vi "Find_Serial_Port.vi"(8 "error in":errorcluster) -> (0 "error out":errorcluster, 3 "Array":string[](array[string]))   [LabVIEW 2011]
doc: "This VI finds the VISA Resource Names of all COM ports on the host machine. It first finds the VISA Resource Names of all serial ports and then filters through these to find which of those are COM ports."
panel:
  out "Resource Names of All COM Devices Found":string[](array[string])
  out "Number of COM Resources Found":i32
  # "Find VISA COM Resource Names:\nThis VI finds the VISA Resource Names of all\nCOM ports on the host machine.  Just run the VI\nto find how many COM ports are found and to\nobtain an array of their VISA Resource Names."
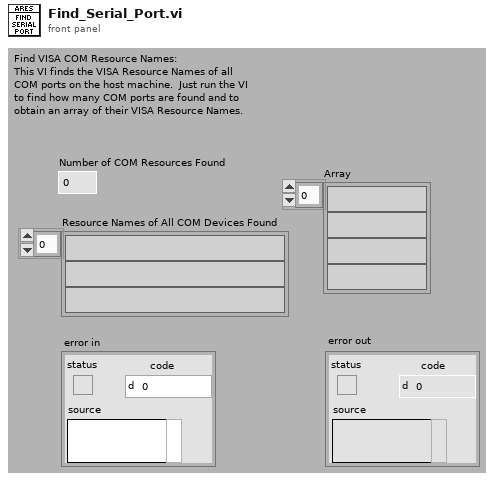
[diagram p1: front panel]
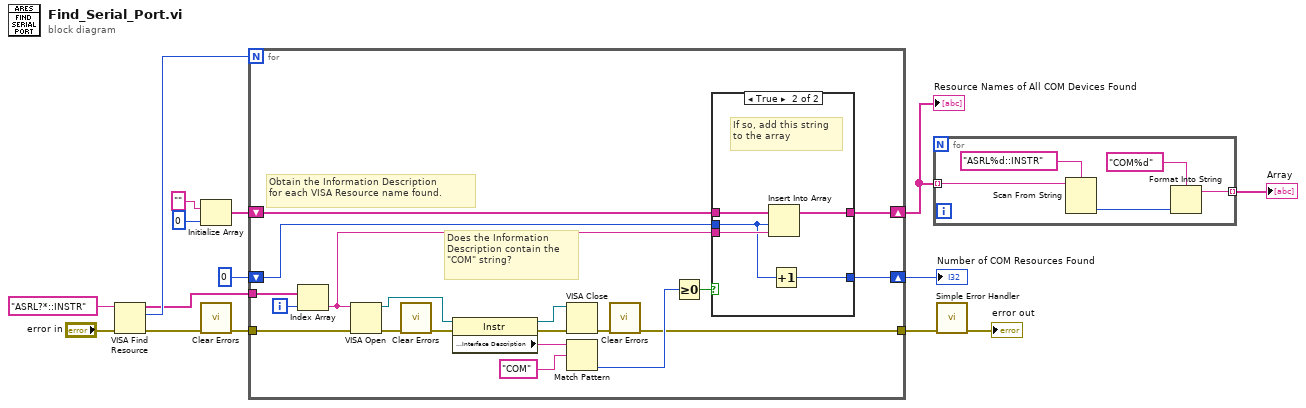
[diagram p0: block diagram]
diagram:
  n1 = VISA Find Resource(8:"error in", 11:"ASRL?*::INSTR" ("expression (\"\")")) -> (0:w9:errorcluster, 2:w14:u32, 3:w13:string[])  [unwired: 1 in]
  n2 = Initialize Array("", 0 ("dimension size")) -> (w10:string[])
  n3 = call <vilib>:"Clear Errors.vi"("error in (no error)"=w9) -> ("error out"=w1:errorcluster)  [unwired: 6 in]
  n4 = for {
    N: w14 -> [_]
    tunnel: w13 -> [w31]
    shift-right: [w23] -> w3
    shift-left: w10 -> [w26]
    tunnel: w1 -> [w22]
    tunnel: [w16] -> w8
    shift-right: [w19] -> w4
    shift-left: 0 -> [w20]
    i -> [w27]
    # "Obtain the Information Description\nfor each VISA Resource name found."
    # "Does the Information \nDescription contain the\n\"COM\" string?"
    n5 = Index Array(array=w31, index=w27) -> (element=w24:string)
    n6 = VISA Open(error in (no error)=w22, VISA resource name=w24) -> (VISA resource name=w25:refnum<visa-resource-name>, error out=w33:errorcluster)  [unwired: 3 in]
    n7 = call <vilib>:"Clear Errors.vi"("error in (no error)"=w33) -> ("error out"=w17:errorcluster)  [unwired: 6 in]
    n8 = property class="Instr"(reference=w25, error in=w17) -> (reference out=w34:refnum<visa-resource-name>, error out=w32:errorcluster, "Interface Information:Interface Description"=w18:string)
    n9 = VISA Close(VISA resource name=w34, error in (no error)=w32) -> (error out=w21:errorcluster)
    n10 = Match Pattern(string=w18, regular expression="COM") -> (offset past match=w29:i32)  [unwired: 1 in, 3 out]
    n11 = call <vilib>:"Clear Errors.vi"("error in (no error)"=w21) -> ("error out"=w16:errorcluster)  [unwired: 6 in]
    n12 = Greater Or Equal To 0?(x=w29) -> (x >= 0?=w28:bool)
    n13 = case shown="True" w28 {
      tunnel: w20 -> [w35 w38]
      tunnel: [w36 w41] -> w23
      tunnel: w26 -> [w36 w40]
      tunnel: w24 -> [_ w39]
      tunnel: [w35 w37] -> w19
      frame False {
        # "If not, do nothing."
      }
      frame True {
        # "If so, add this string\nto the array"
        n14 = Insert Into Array(array=w40, index=w38, new element=w39) -> (w41:string[])
        n15 = Increment(x=w38) -> (x+1=w37:i32)
      }
    }
  }
  "Number of COM Resources Found" <- w4
  "Resource Names of All COM Devices Found" <- w3
  n16 = for {
    tunnel: w3 -> [w43] mode=indexing
    tunnel: [w42] -> w2 mode=indexing
    n17 = Scan From String(format string="ASRL%d::INSTR", input string=w43) -> (output 1=w44:i32)  [unwired: 3 in, 3 out]
    n18 = Format Into String(format string="COM%d" ("regular expression"), w44) -> (resulting string=w42:string)  [unwired: 2 in, 1 out]
  }
  "Array" <- w2
  n19 = call <vilib>:"Simple Error Handler.vi"("error in (no error)"=w8) -> ("error out"=→"error out":errorcluster)  [unwired: 4 in, 4 out]
